vi "OC_read_ind_core.vi"(10 "base":u8 format="%02x") -> (3 "addr":u16)   [LabVIEW 2018]
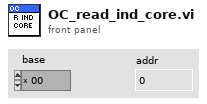
[diagram p1: front panel]
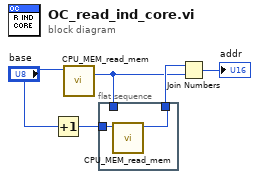
[diagram p0: block diagram]
diagram:
  n1 = Increment(x="base") -> (x+1=w5:u8)
  n2 = call "CPU_MEM_read_mem.vi"("address"="base") -> ("value out"=w1:u8)  [unwired: 10 in]
  n3 = flat-sequence {
    tunnel: w5 -> [w7]
    tunnel: [w6] -> w3
    tunnel: w1 -> [_]
    frame #0 {
      n4 = call "CPU_MEM_read_mem.vi"("address"=w7) -> ("value out"=w6:u8)  [unwired: 10 in]
    }
  }
  n5 = Join Numbers(hi=w3, lo=w1) -> ((hi.lo)=→"addr":u16)
